vi "niRFUtil RFHS Channelizer ClearChannelizer CSG phaseII.vi"(0 "Channelizer Ref":refnum<data-value>, 11 "error in (no error)":errorcluster) -> (4 "Data Left":csg[](array[numeric]), 6 "Channel Data Len":u32[](array[numeric]), 15 "error out":errorcluster)   [LabVIEW 2015, in "niRFUtil.lvlib"]
uses:
  niRFUtil.lvlib
  Includes/niRFUtil RFHS Channelizer ChannelizerInfo CSG.ctl
  Includes/niRFUtil RFHS Channelizer FilterRef.ctl
  Includes/niRFUtil RFHS Channelizer ChannelizerBufferingMode.ctl
  Utilities/Data FIFO/niRFUtil RFHS FIFO Reference.ctl
  Utilities/Data FIFO/niRFUtil RFHS FIFO.ctl
  Includes/niRFUtil RFHS Channelizer ChannelizerType.ctl
  Includes/niRFUtil RFHS Channelizer ChannelizerFlags.ctl
  niRFUtil RFHS Channelizer ChannelizerHandleDllError.vi
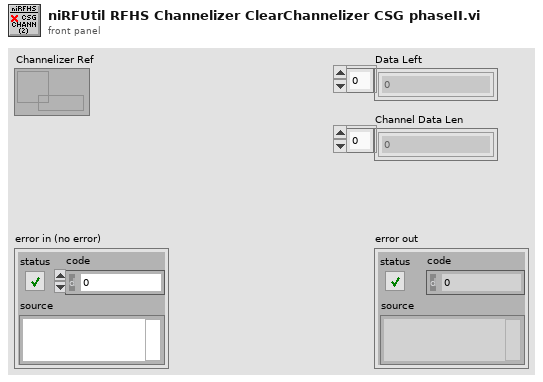
[diagram p1: front panel]
types:
  T1 = typedef "niRFUtil.lvlib/niRFUtil RFHS Channelizer ChannelizerInfo CSG.ctl" = cluster{"Filter LVRef":T2, "Mode":T3, "History":csg[], "Buffer":csg[], "FIFO":T4, "History Len":u32, "Float Cache":csg[], "Double Cache":cdb[], "Type":T6, "Resample Phase":dbl, "fft1Descriptors":u64[], "fft2Descriptors":u64[], "FFT tBuf":csg[], "guardBandLen":i32, "FFT History":csg[], "FFT History Len":u32, "FFTInitDone":u32, "FFT Filter LVRefs":T2[], "FFT fc Offs":u32[], "fft2Sizes":u32[], "BufferW":u32[], "BufferR":u32[], "Buff Off":u32[], "Phase0 (fshift)":dbl[], "Phase (fshift)":dbl[], "fs phase step":dbl[], "Resample Step":dbl, "Flags":T7, "Reset Cnt":i64, "Filter Pass":u32, "Stages":variant[]}
  T2 = typedef "niRFUtil.lvlib/niRFUtil RFHS Channelizer FilterRef.ctl" = cluster{"Ref":u64, "GUID":u64, "Upsample":i32, "Downsample":i32, "Size":i32, "Num Taps":i32}
  T3 = typedef "niRFUtil.lvlib/niRFUtil RFHS Channelizer ChannelizerBufferingMode.ctl" = enum32{"Unbuffered", "Finite", "Continuous"}
  T4 = typedef "niRFUtil.lvlib/niRFUtil RFHS FIFO Reference.ctl" = cluster{"Read Lock":refnum<data-value>, "Info":T5, "Write Lock":refnum<data-value>}
  T5 = typedef "niRFUtil.lvlib/niRFUtil RFHS FIFO.ctl" = cluster{"ID":u64, "Length":u32}
  T6 = typedef "niRFUtil.lvlib/niRFUtil RFHS Channelizer ChannelizerType.ctl" = enum32{"Auto", "Frequency Shift Only", "Resampler Only"}
  T7 = typedef "niRFUtil.lvlib/niRFUtil RFHS Channelizer ChannelizerFlags.ctl" = u32
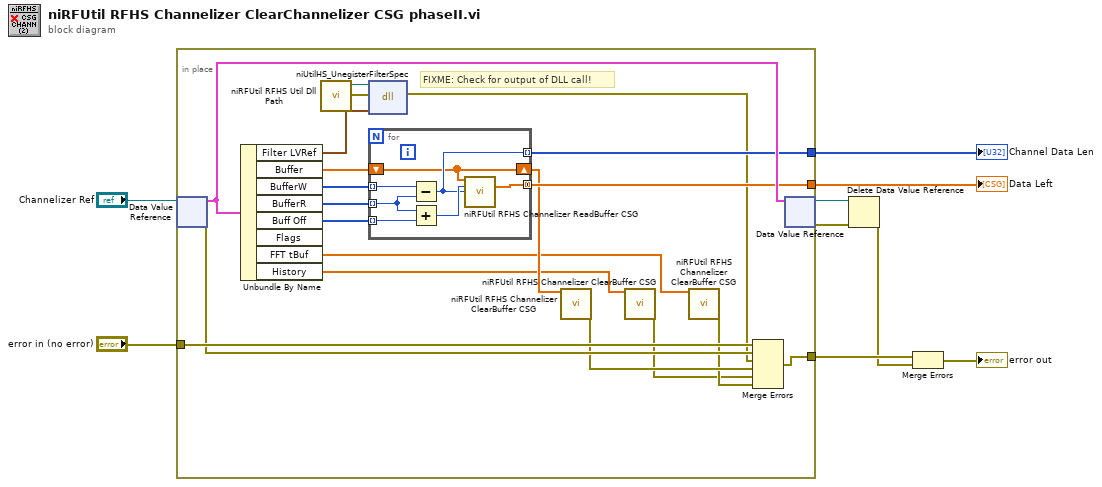
[diagram p0: block diagram]
diagram:
  n1 = in-place {
    in-place-border: [w25] -> w7
    in-place-border: [w23] -> w6
    in-place-border: "error in (no error)" -> [w17]
    in-place-border: [w12] -> w4
    # "FIXME: Check for output of DLL call!"
    n2 = in-place-dvr #1("Channelizer Ref") -> (w27:T1, w16:errorcluster)
    n3 = Unbundle By Name(w27) -> ("Filter LVRef"=w28:T2, "Buffer"=w26:csg[], "BufferW"=w21:u32[], "BufferR"=w20:u32[], "Buff Off"=w24:u32[], "FFT tBuf"=w19:csg[], "History"=w18:csg[])  [unwired: 1 out]
    n4 = call "niRFUtil RFHS Util Dll Path.vi"() -> ("error out"=w10:errorcluster, "Path"=w29:path)  [unwired: 7 in, 3 out]
    n5 = dll-call lib="?" fn="niUtilHS_UnegisterFilterSpec"(path in=w29, error in=w10, "lvRef"=w28) -> (error out=w11:errorcluster)  [unwired: 3 in, 1 out]
    n6 = for {
      tunnel: w21 -> [w36] mode=indexing
      tunnel: w20 -> [w35] mode=indexing
      tunnel: [w31] -> w25 mode=concatenating
      tunnel: w24 -> [w34] mode=indexing
      tunnel: [w32] -> w23 mode=indexing
      shift-right: [w30] -> w22
      shift-left: w26 -> [w30]
      n7 = Subtract(x=w36, y=w35) -> (x-y=w32:u32)
      n8 = Add(x=w35, y=w34) -> (x+y=w33:u32)
      n9 = call "niRFUtil RFHS Channelizer ReadBuffer CSG.vi"("Buffer"=w30, "Index"=w33, "Length"=w32) -> ("Data"=w31:csg[])  [unwired: 12 in]
    }
    n10 = call "niRFUtil RFHS Channelizer ClearBuffer CSG.vi"("Buffer"=w22) -> ("error out"=w15:errorcluster)  [unwired: 14 in]
    n11 = call "niRFUtil RFHS Channelizer ClearBuffer CSG.vi"("Buffer"=w18) -> ("error out"=w13:errorcluster)  [unwired: 14 in]
    n12 = call "niRFUtil RFHS Channelizer ClearBuffer CSG.vi"("Buffer"=w19) -> ("error out"=w14:errorcluster)  [unwired: 14 in]
    n13 = Merge Errors(w17, w16, w11, w15, w13, w14) -> (w12:errorcluster)
    n14 = in-place-dvr #1(w27) -> (w8:refnum<data-value>, w2:errorcluster)
  }
  "Data Left" <- w7
  "Channel Data Len" <- w6
  n15 = Delete Data Value Reference(data value reference=w8, error in=w2) -> (error out=w3:errorcluster)  [unwired: 1 out]
  n16 = Merge Errors(w4, w3) -> (→"error out":errorcluster)
